vi "RT Loop - Low Speed.vi"(11 "Message Queue":refnum<queue>) -> ()   [LabVIEW 2018]
doc: "This RSI Low Speed Loop VI acquires temperature data and digital inputs, and updates digital outputs."
uses:
  Support/Message Queue/Message Cluster.ctl
  Support/Message Queue/Message.ctl
  <vilib>/Platform/TimedLoop/XDataNode/timing_clust.ctl
  <vilib>/Platform/TimedLoop/XDataNode/nitl_modes.ctl
  <vilib>/Platform/TimedLoop/XDataNode/wakeup.ctl
  Controls/VTF Sensors.ctl
  <vilib>/Platform/TimedLoop/XDataNode/loadnilvce.vi
  <vilib>/Platform/TimedLoop/XDataNode/XDataNode.xnode
  <vilib>/Platform/TimedLoop/XDataNode/XDNodeRunTimeDep.lvlib
  support/Message Queue/Message Queue.lvlib
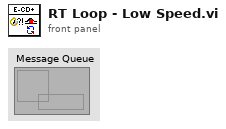
[diagram p1: front panel]
types:
  T1 = typedef "XDNodeRunTimeDep.lvlib/timing_clust.ctl" = cluster{"Expected End [f-1]":u64, "Actual End [f-1]":u64, "Finished Late? [f-1]":bool, "Expected End [i-1]":u64, "Actual End [i-1]":u64, "Finished Late? [i-1]":bool, "Expected Start [i]":u64, "Actual Start [i]":u64, "Expected Start [f]":u64, "Actual Start [f]":u64, "Source Name":string, "Structure Name":string, "Period":i64, "Deadline":i64, "Offset":i64, "Start":i64, "Priority":i32, "Timeout":i32, "Mode":T2, "Wakeup Reason":T3, "Error":errorcluster, "Source Type":string, "Secondary Source Type":string, "Global End Time":u64, "Global Start Time":u64, "Frame Duration":u64, "Iteration Duration":u64, "Assigned CPU":i32, "I/O Scan Engine Mode":u32}
  T2 = typedef "XDNodeRunTimeDep.lvlib/nitl_modes.ctl" = enum32{"No Change", "Process missed periods, maintain original phase", "Discard missed periods, maintain original phase", "Process missed periods, ignore original phase", "Discard missed periods, ignore original phase"}
  T3 = typedef "XDNodeRunTimeDep.lvlib/wakeup.ctl" = enum32{"Normal", "Aborted", "Asynchronous wakeup", "Timing source error", "Timed loop error", "Timeout"}
  T4 = typedef "VTF Sensors.ctl" = cluster{"TJM Temp":dbl, "BrgM Temp":dbl, "Ambient Temp":dbl, "Vessel Temp":dbl}
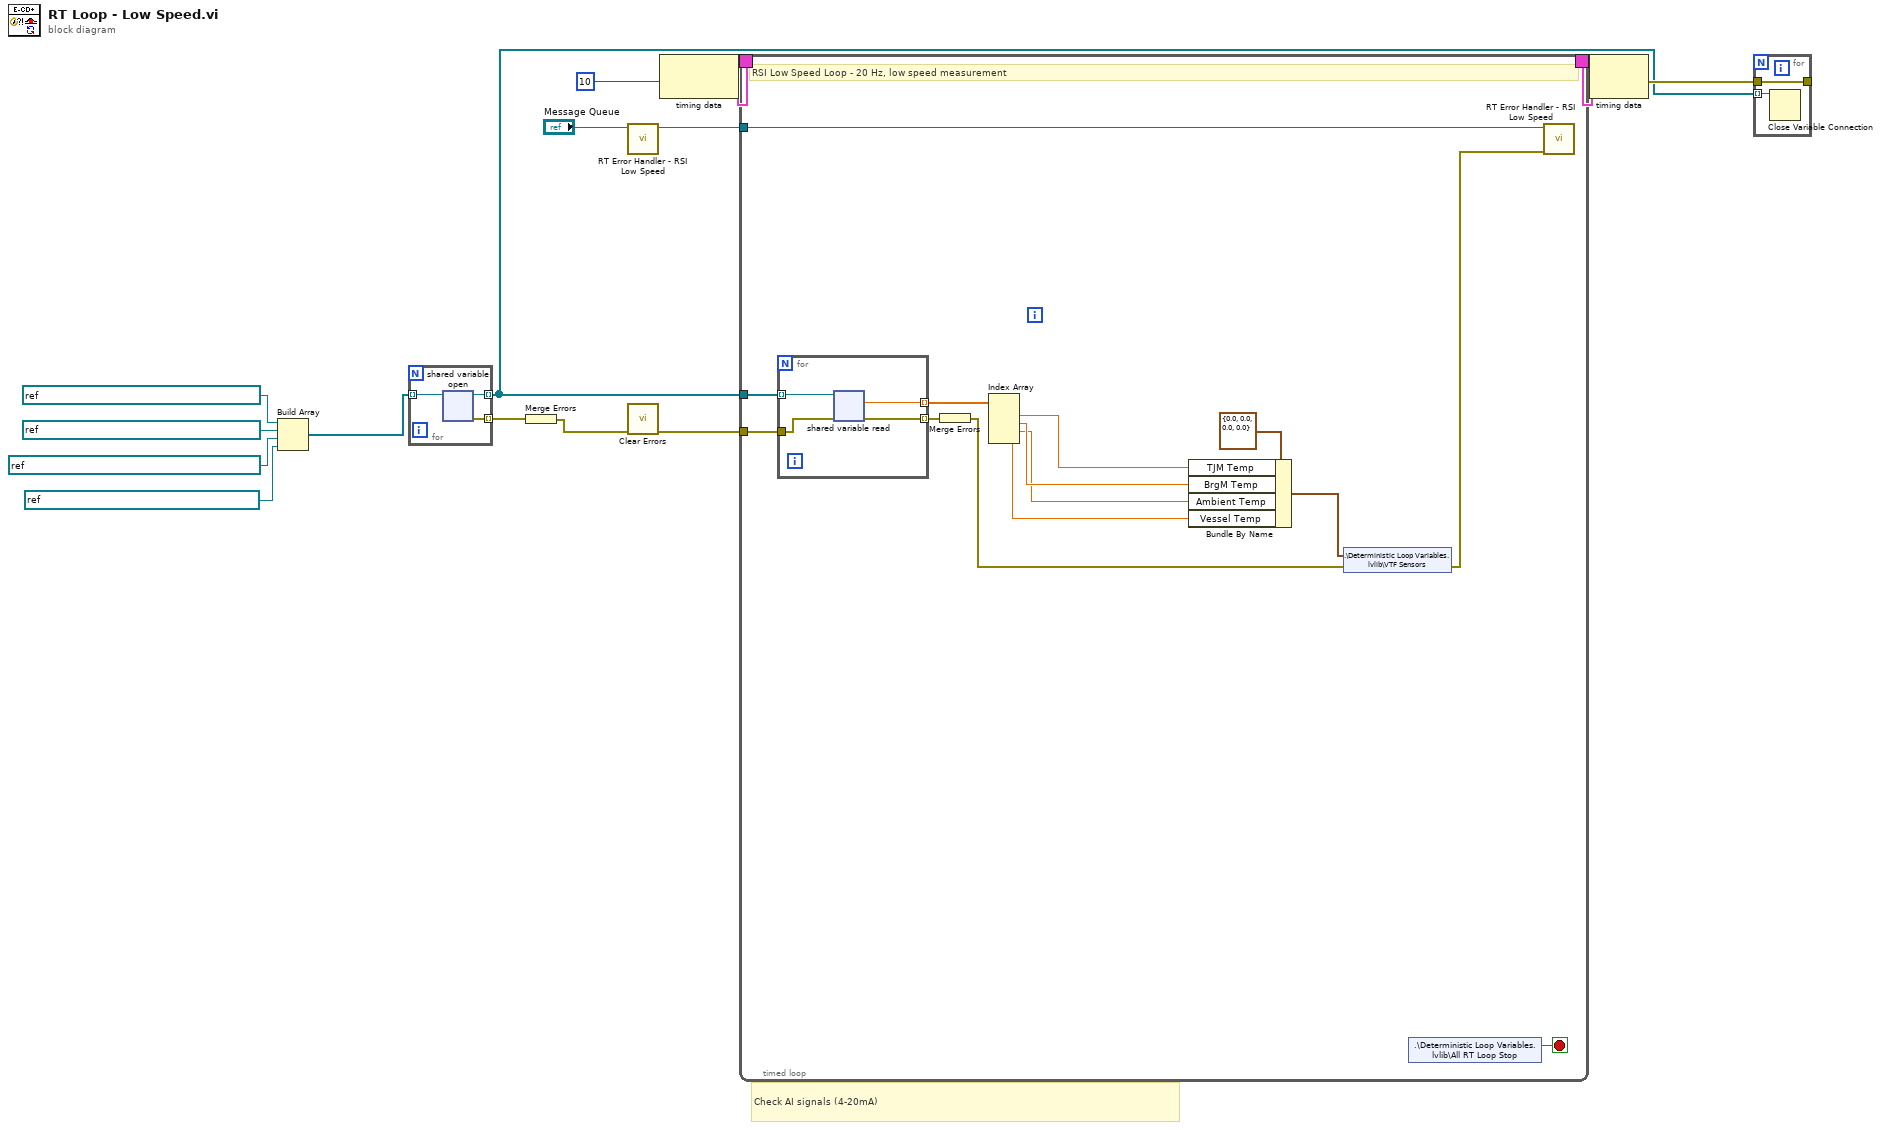
[diagram p0: block diagram]
diagram:
  # "Check AI signals (4-20mA)"
  n1 = Build Array(refnum<k21> "ni.var.io://192.168.1.2/01AI/00TJMTemp" ("shared variable refnum in"), refnum<k21> "ni.var.io://192.168.1.2/01AI/07BRGTemp" ("shared variable refnum in"), refnum<k21> "ni.var.io://192.168.1.2/01AI/01AMBInTemp" ("shared variable refnum in"), refnum<k21> "ni.var.io://192.168.1.2/01AI/02VSLTemp" ("shared variable refnum in")) -> (w4:refnum<k21>[])
  n2 = for {
    tunnel: w4 -> [w18] mode=indexing
    tunnel: [w17] -> w7 mode=indexing
    tunnel: [w16] -> w9 mode=indexing
    n3 = shared-variable-open(w18) -> (w17:refnum<k21>, w16:errorcluster)  [unwired: 1 in]
  }
  n4 = Merge Errors(w9) -> (w10:errorcluster)
  n5 = call "RT Error Handler - RSI Low Speed.vi"("Message Queue"="Message Queue") -> ("dup Message Queue"=w6:refnum<queue>)  [unwired: 9 in, 1 out]
  n6 = call <vilib>:"Clear Errors.vi"("error in (no error)"=w10) -> ("error out"=w8:errorcluster)  [unwired: 5 in, 1 out]
  n7 = node-c288(i64 10 ("Period")) -> (w15:T1)
  n8 = timed-loop {
    timing: w15 -> [_]
    timing-out: [_] -> w14
    tunnel: w6 -> [w31]
    tunnel: w8 -> [w28]
    tunnel: w7 -> [w27]
    stop <- w32 stop-if-true
    # "RSI Low Speed Loop - 20 Hz, low speed measurement"
    n9 = for {
      tunnel: w28 -> [w35]
      tunnel: w27 -> [w36] mode=indexing
      tunnel: [w34] -> w26 mode=indexing
      tunnel: [w33] -> w24 mode=indexing
      n10 = shared-variable-read(w36, w35) -> (w33:errorcluster, w34:dbl)  [unwired: 1 out]
    }
    n11 = Merge Errors(w24) -> (w22:errorcluster)
    n12 = Index Array(array=w26) -> (element #1=w25:dbl, element #2=w23:dbl, element #3=w20:dbl, element #4=w19:dbl)  [unwired: 4 in]
    n13 = Bundle By Name(cluster=T4 {"TJM Temp"=0.0, "BrgM Temp"=0.0, "Ambient Temp"=0.0, "Vessel Temp"=0.0} ("HPU Sensors"), "TJM Temp"=w25, "BrgM Temp"=w23, "Ambient Temp"=w20, "Vessel Temp"=w19) -> (w29:T4)
    n14 = shared-variable ".\\Deterministic Loop Variables.lvlib\\VTF Sensors"(w29, error in=w22) -> (error out=w21:errorcluster)
    n15 = shared-variable ".\\Deterministic Loop Variables.lvlib\\All RT Loop Stop"() -> (w32:bool)  [unwired: 1 in, 1 out]
    n16 = call "RT Error Handler - RSI Low Speed.vi"("error in (no error)"=w21, "Message Queue"=w31) -> ()  [unwired: 8 in, 2 out]
  }
  n17 = node-c288(w14) -> (w12:errorcluster)
  n18 = for {
    tunnel: w7 -> [w40] mode=indexing
    tunnel: w12 -> [w39]
    tunnel: [w39] -> _
    n19 = Close Variable Connection(11:w40) -> ()  [unwired: 1 in, 1 out]
  }
